vi "Istwerte verarbeiten Regler.vi"(8 "error in (no error)":errorcluster caption="Fehler (Eingang, kein Fehler)", 9 "Index":u16, 10 "Istwerte":u16[](array[numeric]), 11 "Schneider Steuerung PNS Eingang":refnum<class "Schneider Steuerung PNS.lvclass">) -> (0 "error out":errorcluster caption="Fehler (Ausgang)", 3 "Schneider Steuerung PNS Ausgang":refnum<class "Schneider Steuerung PNS.lvclass">)   [LabVIEW 2020, in "Schneider Steuerung PNS.lvclass"]
uses:
  Schneider Steuerung PNS.lvclass
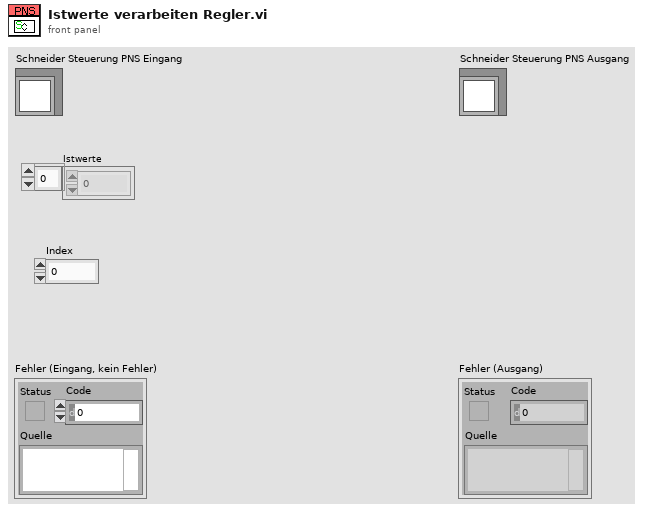
[diagram p1: front panel]
types:
  T1 = typedef "Steuerung PNS.lvclass/Regler.ctl" = cluster{"Istwert":i16, "Sollwert":i16, "Alarm MIN":i16, "Alarm MAX":i16, "Regler sperren":i16, "Analog Ausgang":i16}[]
  T2 = cluster{"Istwerte[0]":u16, "Istwerte[1]":u16, "Istwerte[2]":u16, "Istwerte[3]":u16, "Istwerte[4]":u16, "Istwerte[5]":u16}
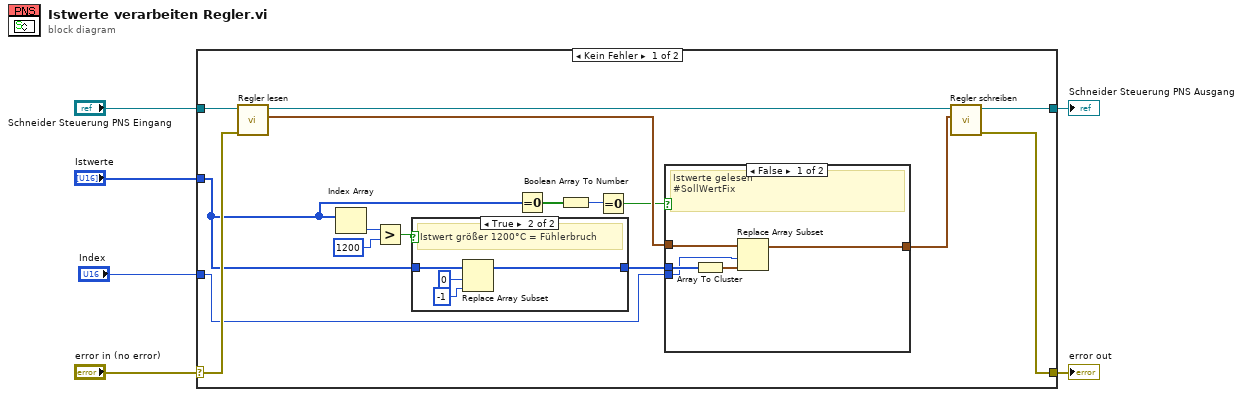
[diagram p0: block diagram]
diagram:
  n1 = case shown="Kein Fehler" "error in (no error)" {
    selector: "error in (no error)" -> [w19 w35]
    tunnel: [w18 w35] -> w5
    tunnel: [w20 w34] -> w3
    tunnel: "Schneider Steuerung PNS Eingang" -> [w22 w34]
    tunnel: "Istwerte" -> [w10 _]
    tunnel: "Index" -> [w12 _]
    frame No Error {
      n2 = call-dynamic "Regler lesen.vi"("error in (no error)"=w19, "Steuerung PNS (Eingang)"=w22) -> ("Regler"=w14:T1, "Steuerung PNS (Ausgang)"=w21:refnum<class "Schneider Steuerung PNS.lvclass">)  [unwired: 7 in, 1 out]
      n3 = Index Array(array=w10) -> (element=w16:u16)  [unwired: 1 in]
      n4 = Greater?(x=w16, y=i16 1200) -> (0:w15:bool)
      n5 = case shown="True" w15 {
        tunnel: w10 -> [w29 w30]
        tunnel: [w29 w33] -> w13
        frame False {
        }
        frame True {
          # "Istwert größer 1200°C = Fühlerbruch"
          n6 = Replace Array Subset(array=w30, new element=i16 -1 ("Neues Element/Teil-Array"), index=0 ("Index")) -> (w33:u16[])
        }
      }
      n7 = Equal To 0?(x=w10) -> (x = 0?=w9:bool[])
      n8 = Boolean Array To Number(Boolean array=w9) -> (number=w8:u32)
      n9 = Equal To 0?(x=w8) -> (x = 0?=w7:bool)
      n10 = case shown="False" w7 {
        tunnel: w14 -> [w26 w28]
        tunnel: w13 -> [w25 _]
        tunnel: w12 -> [w24 _]
        tunnel: [w23 w28] -> w11
        frame False {
          # "Istwerte gelesen \n#SollWertFix"
          n11 = Array To Cluster(array=w25) -> (cluster=w27:T2)
          n12 = Replace Array Subset(array=w26, new element=w27, index=w24) -> (w23:T1)
        }
        frame True {
          # "Istwert = 0\nWerte wurden wahrscheinlich\nnicht gelesen!!!!"
        }
      }
      n13 = call-dynamic "Regler schreiben.vi"("Regler"=w11, "Steuerung PNS (Eingang)"=w21) -> ("error out"=w18:errorcluster, "Steuerung PNS (Ausgang)"=w20:refnum<class "Schneider Steuerung PNS.lvclass">)  [unwired: 8 in]
    }
    frame Error {
    }
  }
  "error out" <- w5
  "Schneider Steuerung PNS Ausgang" <- w3
